vi "S7 Optimized Read Cluster Array.vi"(7 "Optimized Data Index":T1[](array[typedef]) {"Bit Number" max=7 step=1}, 8 "error in":errorcluster, 9 "S7 Optimized Read Array":T3[](array[typedef]) {"Address Areas" items=["I/O (P)"=128, "Input (I)"=129, "Output (Q)"=130, "Bit Memory (M)"=131, "Data (DB)"=132, "Instance Data (DI)"=133, "Local Data (L)"=134, "Predecessor Local Data (VL)"=135]; "Read / Write" items=["Read"=4, "Write"=5]; "Bit Number / Byte Length" max=7 step=1}, 10 "Timeout":u32, 11 "TCP Connection Ref":refnum<k5>) -> (0 "error out":errorcluster, 1 "Data Valid Array":bool[](array[boolean]), 2 "Output Data":dbl[](array[numeric]), 3 "TCP Connection Ref Out":refnum<k5>)   [LabVIEW 2017, in "S7 TCP.lvlib"]
uses:
  S7 TCP.lvlib
  S7 Read Write Cluster.ctl
  Data Type.ctl
  Optimized Data Index.ctl
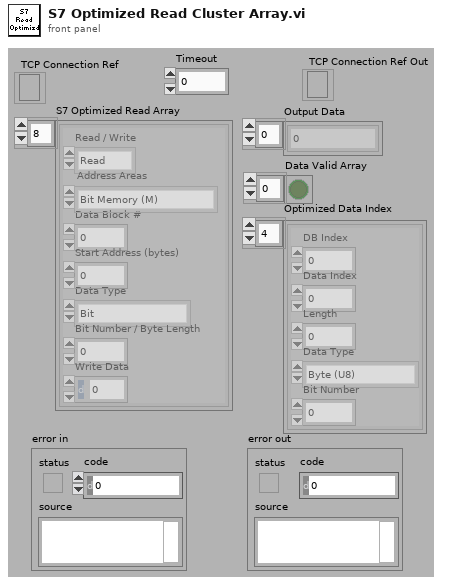
[diagram p1: front panel]
types:
  T1 = typedef "S7 TCP.lvlib/Optimized Data Index.ctl" = cluster{"DB Index":i32, "Data Index":i32, "Length":i32, "Data Type":T2, "Bit Number":u8}
  T2 = typedef "S7 TCP.lvlib/Data Type.ctl" = enum16{"Bit", "Byte (U8)", "Signed Byte (I8)", "Word (U16)", "Signed Word (I16)", "Long (U32)", "Signed Long (I32)", "Real (SGL)", "Defined Byte Length"}
  T3 = typedef "S7 TCP.lvlib/S7 Read Write Cluster.ctl" = cluster{"Read / Write":u8, "Address Areas":u8, "Data Block #":u16, "Start Address (bytes)":u32, "Data Type":T2, "Bit Number / Byte Length":u8, "Write Data":dbl}
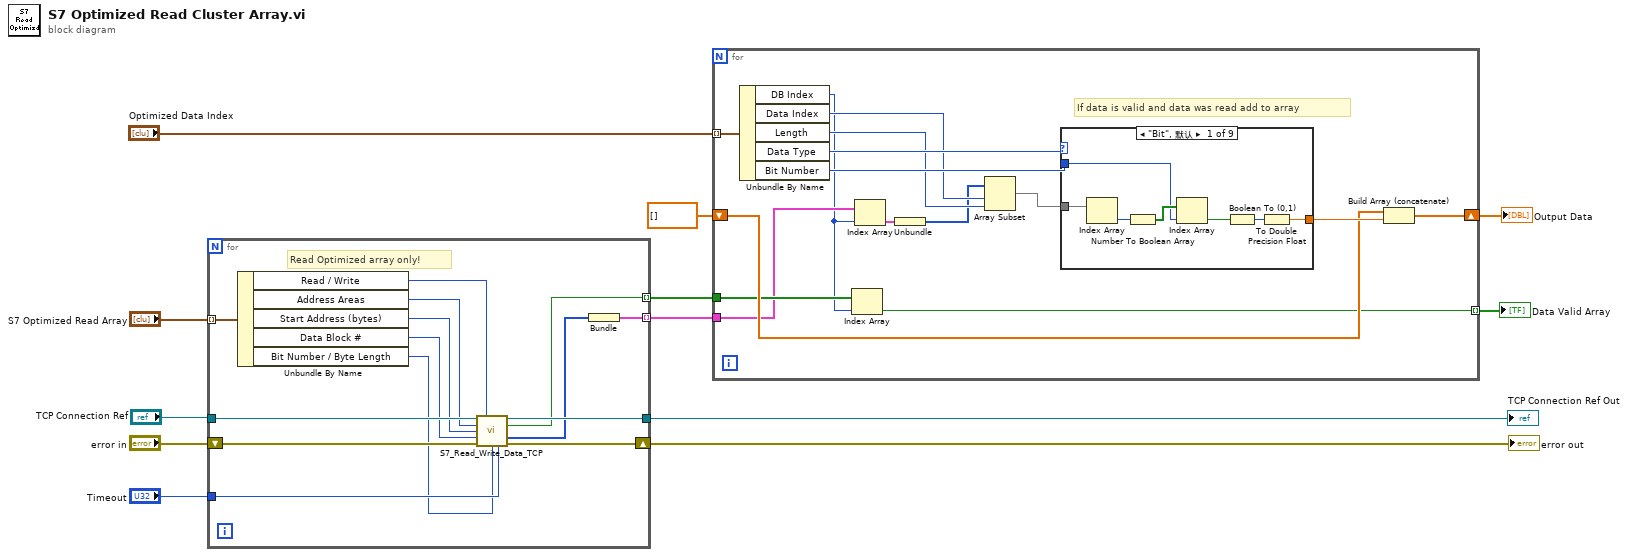
[diagram p0: block diagram]
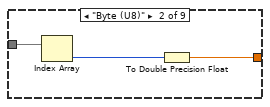
[diagram p2: hidden frame]
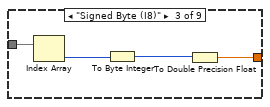
[diagram p3: hidden frame]
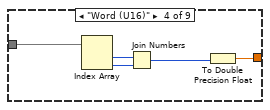
[diagram p4: hidden frame]
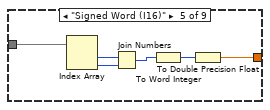
[diagram p5: hidden frame]
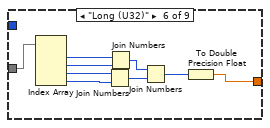
[diagram p6: hidden frame]
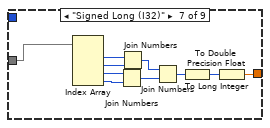
[diagram p7: hidden frame]
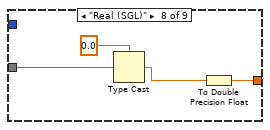
[diagram p8: hidden frame]
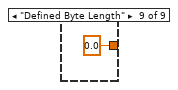
[diagram p9: hidden frame]
diagram:
  n1 = for {
    tunnel: "Timeout" -> [w17]
    tunnel: "TCP Connection Ref" -> [w23]
    tunnel: [w25] -> w7
    tunnel: "S7 Optimized Read Array" -> [w24] mode=indexing
    shift-right: [w26] -> w12
    shift-left: "error in" -> [w22]
    tunnel: [w16] -> w3 mode=indexing
    tunnel: [w14] -> w1 mode=indexing
    # "Read Optimized array only!"
    n2 = Unbundle By Name(w24) -> ("Read / Write"=w18:u8, "Address Areas"=w19:u8, "Start Address (bytes)"=w20:u32, "Data Block #"=w21:u16, "Bit Number / Byte Length"=w13:u8)
    n3 = call "S7_Read_Write_Data_TCP.vi"("TCP Connection Ref"=w23, "Read / Write"=w18, "Address Areas"=w19, "Start Address (bytes)"=w20, "Data Block #"=w21, "error in"=w22, "Length (bytes)"=w13, "Timeout"=w17) -> ("TCP Connection Ref Out"=w25:refnum<k5>, "Data Valid"=w16:bool, "Data Read"=w15:u8[], "error out"=w26:errorcluster)  [unwired: 1 in, 3 out]
    n4 = Bundle("Data Read"=w15) -> (w14:cluster{"Data Read":u8[]})  [unwired: 1 in]
  }
  "error out" <- w12
  "TCP Connection Ref Out" <- w7
  n5 = for {
    shift-right: [w39] -> w5
    shift-left: dbl[] [] -> [w40]
    tunnel: w1 -> [w31]
    tunnel: "Optimized Data Index" -> [w38] mode=indexing
    tunnel: w3 -> [w35]
    tunnel: [w34] -> w2 mode=indexing
    # "If data is valid and data was read add to array"
    n6 = Unbundle By Name(w38) -> ("DB Index"=w27:i32, "Data Index"=w33:i32, "Length"=w32:i32, "Data Type"=w37:T2, "Bit Number"=w36:u8)
    n7 = Index Array(array=w35, index=w27) -> (element=w34:bool)
    n8 = Index Array(array=w31, index=w27) -> (element=w30:cluster{"Data Read":u8[]})
    n9 = Unbundle(w30) -> ("Data Read"=w29:u8[])
    n10 = Array Subset(array=w29, index=w33, length=w32) -> (w28:u8[])
    n11 = case shown="\"Bit\", 默认" w37 {
      tunnel: w28 -> [w48 w51 w55 w60 w64 w69 w76 w89 _]
      tunnel: w36 -> [w45 _ _ _ _ _ _ _ _]
      tunnel: [w42 w49 w54 w57 w63 w67 w79 w86 0.0] -> w41
      frame "Bit", Default {
        n12 = Index Array(array=w48) -> (element=w47:u8)  [unwired: 1 in]
        n13 = Number To Boolean Array(number=w47) -> (Boolean array=w46:bool[])
        n14 = Index Array(array=w46, index=w45) -> (element=w44:bool)
        n15 = Boolean To (0,1)(Boolean=w44) -> (0, 1=w43:i16)
        n16 = To Double Precision Float(number=w43) -> (double precision float=w42:dbl)
      }
      frame "Byte (U8)" {
        n17 = Index Array(array=w51) -> (element=w50:u8)  [unwired: 1 in]
        n18 = To Double Precision Float(number=w50) -> (double precision float=w49:dbl)
      }
      frame "Signed Byte (I8)" {
        n19 = Index Array(array=w55) -> (element=w53:u8)  [unwired: 1 in]
        n20 = To Byte Integer(number=w53) -> (8bit integer=w52:i8)
        n21 = To Double Precision Float(number=w52) -> (double precision float=w54:dbl)
      }
      frame "Word (U16)" {
        n22 = Index Array(array=w60) -> (element #1=w58:u8, element #2=w59:u8)  [unwired: 2 in]
        n23 = Join Numbers(hi=w58, lo=w59) -> ((hi.lo)=w56:u16)
        n24 = To Double Precision Float(number=w56) -> (double precision float=w57:dbl)
      }
      frame "Signed Word (I16)" {
        n25 = Index Array(array=w64) -> (element #1=w65:u8, element #2=w66:u8)  [unwired: 2 in]
        n26 = Join Numbers(hi=w65, lo=w66) -> ((hi.lo)=w62:u16)
        n27 = To Word Integer(number=w62) -> (16bit integer=w61:i16)
        n28 = To Double Precision Float(number=w61) -> (double precision float=w63:dbl)
      }
      frame "Long (U32)" {
        n29 = Index Array(array=w69) -> (element #1=w74:u8, element #2=w75:u8, element #3=w71:u8, element #4=w70:u8)  [unwired: 4 in]
        n30 = Join Numbers(hi=w71, lo=w70) -> ((hi.lo)=w72:u16)
        n31 = Join Numbers(hi=w74, lo=w75) -> ((hi.lo)=w73:u16)
        n32 = Join Numbers(hi=w73, lo=w72) -> ((hi.lo)=w68:u32)
        n33 = To Double Precision Float(number=w68) -> (double precision float=w67:dbl)
      }
      frame "Signed Long (I32)" {
        n34 = Index Array(array=w76) -> (element #1=w84:u8, element #2=w85:u8, element #3=w81:u8, element #4=w80:u8)  [unwired: 4 in]
        n35 = Join Numbers(hi=w81, lo=w80) -> ((hi.lo)=w82:u16)
        n36 = Join Numbers(hi=w84, lo=w85) -> ((hi.lo)=w83:u16)
        n37 = Join Numbers(hi=w83, lo=w82) -> ((hi.lo)=w78:u32)
        n38 = To Long Integer(number=w78) -> (32bit integer=w77:i32)
        n39 = To Double Precision Float(number=w77) -> (double precision float=w79:dbl)
      }
      frame "Real (SGL)" {
        n40 = Type Cast(type=sgl 0.0, x=w89) -> (*(type *) &x=w87:sgl)
        n41 = To Double Precision Float(number=w87) -> (double precision float=w86:dbl)
      }
      frame "Defined Byte Length" {
      }
    }
    n42 = Build Array (concatenate)(w40, w41) -> (w39:dbl[])
  }
  "Output Data" <- w5
  "Data Valid Array" <- w2
